vi "resolve control references.vi"(4 "output dictionary":refnum<class "data dictionary.lvclass">, 6 "input dictionary":refnum<class "data dictionary.lvclass">, 8 "error in":errorcluster, 10 "UI Ref":refnum<vi>, 11 "channels in":refnum<class "TBM channel.lvclass">[](array[class])) -> (0 "error out":errorcluster, 2 "indicators":T1[](array[typedef]), 3 "controls":T1[](array[typedef]))   [LabVIEW 2014, in "UI Reference runtime.lvclass"]
uses:
  UI Reference runtime.lvclass
  <vilib>/NI/Tag Bus Module Framework/channel/TBM channel.lvclass
  control index set.ctl
  <vilib>/NI/Tag Bus/tag/Data Type.ctl
  <vilib>/NI/Tag Bus/dictionary/data dictionary.lvclass
  <vilib>/NI/Tag Bus Module Framework/channel/TBM channel.lvclass/TBM channel.ctl
  <vilib>/NI/Tag Bus/tag/tag descriptor.lvclass/tag descriptor.ctl
  <vilib>/NI/Tag Bus Module Framework/channel/Read channel classification.vi
  <vilib>/NI/Tag Bus/tag/read tag name.vi
  <vilib>/NI/Tag Bus/tag/read data type.vi
  <vilib>/ErrorRing/Error Ring.xnode
  <vilib>/NI/Tag Bus/tag/tag descriptor.lvclass
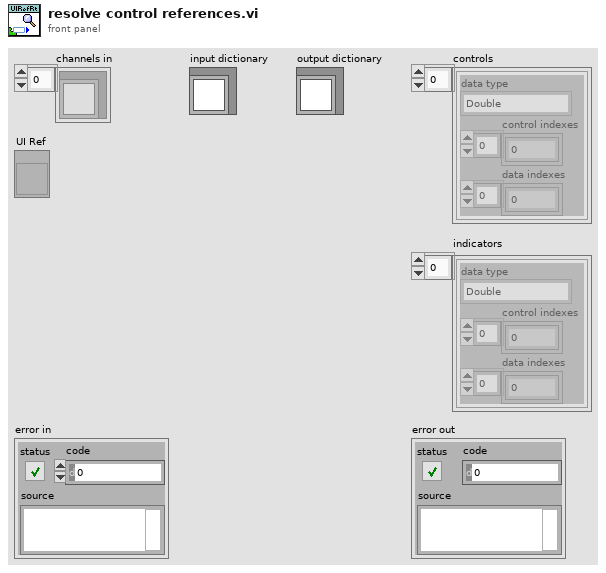
[diagram p1: front panel]
types:
  T1 = typedef "UI Reference runtime.lvclass/control index set.ctl" = cluster{"data type":T2, "control indexes":i32[], "data indexes":i32[]}
  T2 = typedef "tag bus.lvlib/tag descriptor.lvclass/Data Type.ctl" = enum16{"Double", "Single", "I64", "I32", "I16", "I8", "U64", "U32", "U16", "U8", "Boolean", "String", "Array of Double", "Array of Single", "Array of I64", "Array of I32", "Array of I16", "Array of I8", "Array of U64", "Array of U32", "Array of U16", "Array of U8", "Array of Boolean", "Array of String"}
  T3 = typedef "TBM channel.lvclass/channel classification.ctl" = enum16{"input data", "output data", "processing parameter", "processing result"}
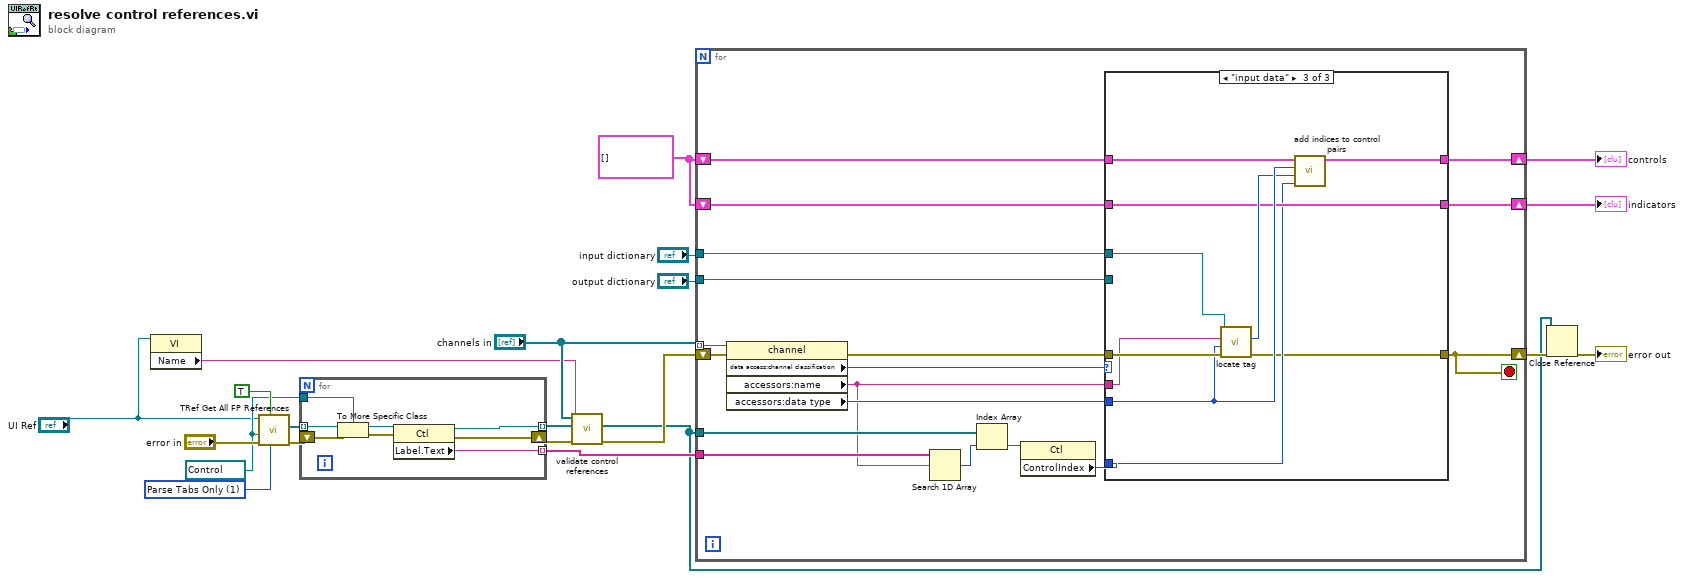
[diagram p0: block diagram]
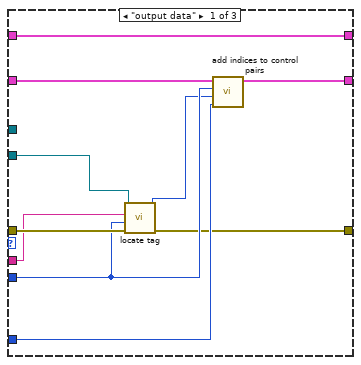
[diagram p2: hidden frame]
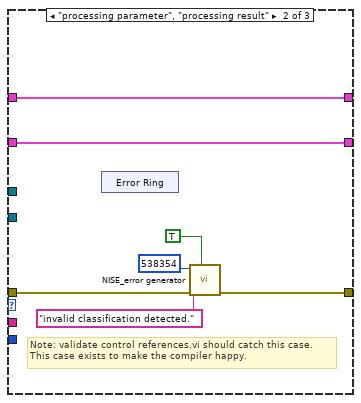
[diagram p3: hidden frame]
diagram:
  w11 = u16 1 items=["Parse All", "Parse Tabs Only"] ("Parsing Rule")
  w9 = refnum<vi> refnum ("Ctl Refnum")
  w20 = T1[] [] ("indicators")
  n1 = property class="VI"(reference="UI Ref") -> ("Name"=w2:string)  [unwired: 1 in, 2 out]
  n2 = call <vilib>:"TRef Get All FP References.vi"("Parsing Rule"=w11, "Ignore Decorations?"=TRUE, "error in (no error)"="error in", "GObj Refnum"=w9, "VI Refnum"="UI Ref") -> ("error out"=w10:errorcluster, "All FP Objects"=w8:refnum<vi>[])  [unwired: 2 in, 3 out]
  n3 = for {
    shift-right: [w28] -> w4
    shift-left: w10 -> [w25]
    tunnel: [w27] -> w5 mode=indexing
    tunnel: [w26] -> w1 mode=indexing
    tunnel: w9 -> [w23]
    tunnel: w8 -> [w22] mode=indexing
    n4 = To More Specific Class(target class=w23, reference=w22, error in=w25) -> (specific class reference=w21:refnum<vi>, error out=w24:errorcluster)
    n5 = property class="Ctl"(reference=w21, error in=w24) -> (reference out=w26:refnum<vi>, error out=w28:errorcluster, "Label.Text"=w27:string)
  }
  n6 = call "validate control references.vi"("error in (no error)"=w4, "VI Name"=w2, "front panel elements in"=w1, "channels in"="channels in") -> ("error out"=w3:errorcluster)  [unwired: 7 in]
  n7 = for {
    tunnel: "channels in" -> [w46] mode=indexing
    tunnel: w1 -> [w32]
    tunnel: w5 -> [w31]
    shift-right: [w41] -> w18
    shift-left: w20 -> [w40]
    shift-right: [w38] -> w17
    shift-left: w20 -> [w39]
    shift-right: [w42] -> w19
    shift-left: w3 -> [w45]
    tunnel: "output dictionary" -> [w35]
    tunnel: "input dictionary" -> [w37]
    stop <- w42 stop-if-true
    n8 = property class="channel"(reference=w46, error in=w45) -> (error out=w43:errorcluster, "data access:channel classification"=w44:T3, "accessors:name"=w30:string, "accessors:data type"=w36:T2)  [unwired: 1 out]
    n9 = Search 1D Array(1D array=w31, element=w30) -> (index of element=w34:i32)  [unwired: 1 in]
    n10 = Index Array(array=w32, index=w34) -> (element=w33:refnum<vi>)
    n11 = property class="Ctl"(reference=w33) -> ("ControlIndex"=w29:i32)  [unwired: 1 in, 2 out]
    n12 = case shown="\"input data\"" w44 {
      tunnel: w43 -> [w56 w60 w74]
      tunnel: [w47 w61 w65] -> w42
      tunnel: [w50 w63 w68] -> w41
      tunnel: w40 -> [w50 w63 w69]
      tunnel: w39 -> [w52 w62 w67]
      tunnel: [w51 w62 w67] -> w38
      tunnel: w37 -> [_ _ w70]
      tunnel: w30 -> [w54 _ w73]
      tunnel: w36 -> [w53 _ w72]
      tunnel: w35 -> [w55 _ _]
      tunnel: w29 -> [w48 _ w66]
      frame "output data" {
        n13 = call <vilib>:"locate tag.vi"("error in"=w56, "data type"=w53, "name"=w54, "data dictionary in"=w55) -> ("error out"=w47:errorcluster, "index"=w49:i32)  [unwired: 5 in, 1 out]
        n14 = call "add indices to control pairs.vi"("control index"=w48, "data index"=w49, "data type"=w53, "pairs in"=w52) -> ("pairs out"=w51:T1[])  [unwired: 7 in]
      }
      frame "processing parameter", "processing result" {
        # "Note: validate control references.vi should catch this case.\nThis case exists to make the compiler happy."
        n15 = xnode "Error Ring"() -> ()  [unwired: 1 out]
        n16 = call <vilib>:"NISE_error generator.vi"("error (T)"=TRUE, "error in"=w60, "append error message"="invalid classification detected.", "error code (0)"=538354) -> ("error out"=w61:errorcluster)  [unwired: 5 in]
      }
      frame "input data" {
        n17 = call <vilib>:"locate tag.vi"("error in"=w74, "data type"=w72, "name"=w73, "data dictionary in"=w70) -> ("error out"=w65:errorcluster, "index"=w71:i32)  [unwired: 5 in, 1 out]
        n18 = call "add indices to control pairs.vi"("control index"=w66, "data index"=w71, "data type"=w72, "pairs in"=w69) -> ("pairs out"=w68:T1[])  [unwired: 7 in]
      }
    }
  }
  "controls" <- w18
  "indicators" <- w17
  n19 = Close Reference(reference=w1, error in (no error)=w19) -> (error out=→"error out":errorcluster)
